vi "Fix BD Size.vi"(8 "error in (no error)":errorcluster, 11 "vi ref":refnum<vi>) -> (0 "error out":errorcluster, 3 "vi ref (dup)":refnum<vi>)   [LabVIEW 2021]
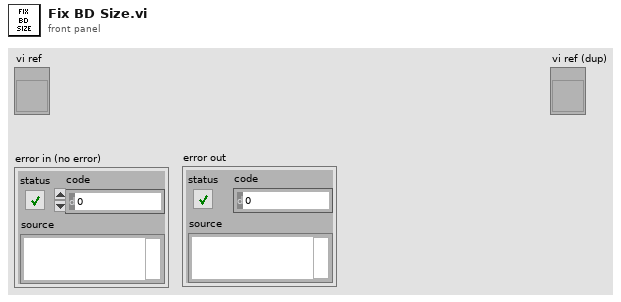
[diagram p1: front panel]
types:
  T1 = cluster{"min x":i32, "min y":i32, "max x":i32, "max y":i32}
  T2 = typedef "LVRectTypeDef.ctl" = cluster{"Left":i16, "Top":i16, "Right":i16, "Bottom":i16}
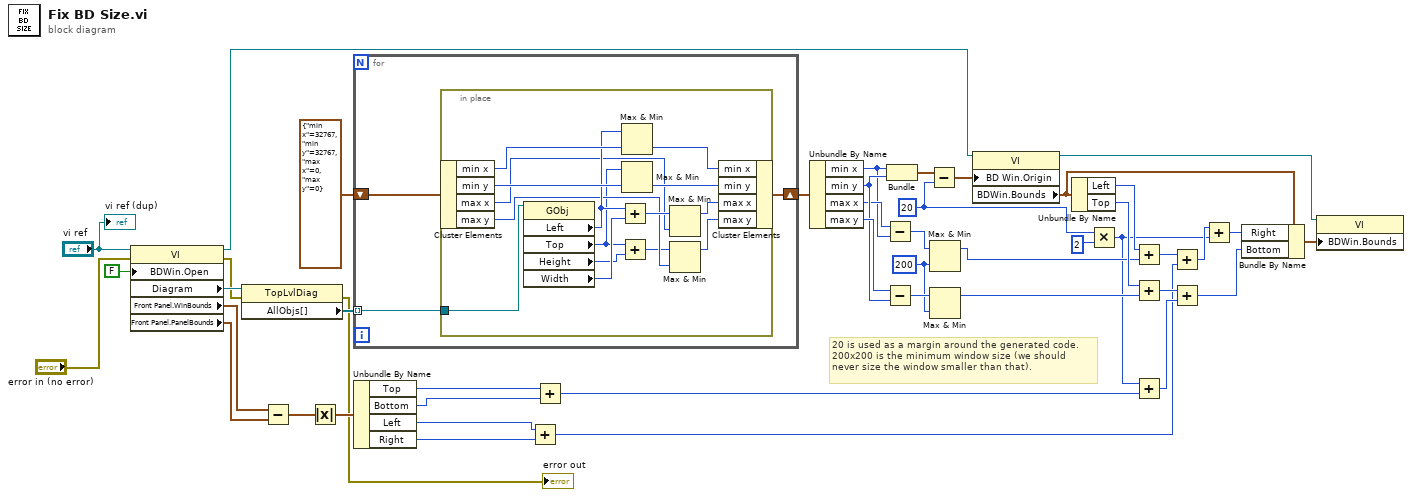
[diagram p0: block diagram]
diagram:
  w11 = 20 ("y")
  w24 = 200 ("y")
  # "20 is used as a margin around the generated code.\n200x200 is the minimum window size (we should\nnever size the window smaller than that)."
  n1 = property class="VI"(reference="vi ref", error in="error in (no error)", "BDWin.Open"=FALSE ("Block Diagram Window:Open")) -> (reference out=w40:refnum<vi>, error out=w2:errorcluster, "Diagram"=w43:refnum<vi>, "Front Panel.WinBounds"=w20:T2, "Front Panel.PanelBounds"=w19:T2)
  n2 = property class="TopLvlDiag"(reference=w43, error in=w2) -> (error out=→"error out":errorcluster, "AllObjs[]"=w42:refnum<vi>[])  [unwired: 1 out]
  n3 = Subtract(x=w20, y=w19) -> (x-y=w9:T2)
  n4 = Absolute Value(x=w9) -> (abs(x)=w8:T2)
  n5 = for {
    tunnel: w42 -> [w47] mode=indexing
    shift-right: [w46] -> w39
    shift-left: T1 {"min x"=32767, "min y"=32767, "max x"=0, "max y"=0} -> [w48]
    n6 = in-place {
      in-place-border: w47 -> [w63]
      n7 = in-place-cluster #1(w48) -> ("min x"=w62:i32, "min y"=w60:i32, "max x"=w55:i32, "max y"=w53:i32)
      n8 = property class="GObj"(reference=w63) -> ("Left"=w58:i32, "Top"=w52:i32, "Height"=w51:u32, "Width"=w57:u32)  [unwired: 1 in, 2 out]
      n9 = Add(x=w58, y=w57) -> (x+y=w56:u32)
      n10 = Add(x=w52, y=w51) -> (x+y=w50:u32)
      n11 = Max & Min(x=w58, y=w62) -> (min(x,y)=w61:i32)  [unwired: 1 out]
      n12 = Max & Min(x=w52, y=w60) -> (min(x,y)=w59:i32)  [unwired: 1 out]
      n13 = Max & Min(x=w56, y=w55) -> (max(x,y)=w54:u32)  [unwired: 1 out]
      n14 = Max & Min(x=w50, y=w53) -> (max(x,y)=w49:u32)  [unwired: 1 out]
      n15 = in-place-cluster #1("min x"=w61, "min y"=w59, "max x"=w54, "max y"=w49) -> (w46:T1)
    }
  }
  n16 = Unbundle By Name(w8) -> ("Top"=w7:i16, "Bottom"=w6:i16, "Left"=w5:i16, "Right"=w4:i16)
  n17 = Add(x=w5, y=w4) -> (x+y=w15:i16)
  n18 = Add(x=w7, y=w6) -> (x+y=w17:i16)
  n19 = Unbundle By Name(w39) -> ("min x"=w35:i32, "min y"=w37:i32, "max x"=w36:i32, "max y"=w38:i32)
  n20 = Subtract(x=w36, y=w35) -> (x-y=w27:i32)
  n21 = Subtract(x=w38, y=w37) -> (x-y=w25:i32)
  n22 = Bundle("min x"=w35, "min y"=w37) -> (w22:cluster{"min x":i32, "min y":i32})  [unwired: 1 in]
  n23 = Subtract(x=w22, y=w11) -> (x-y=w21:cluster{"min x":i32, "min y":i32})
  n24 = Max & Min(x=w27, y=w24) -> (max(x,y)=w26:i32)  [unwired: 1 out]
  n25 = Max & Min(x=w25, y=w24) -> (max(x,y)=w23:i32)  [unwired: 1 out]
  n26 = property class="VI"(reference=w40, "BD Win.Origin"=w21) -> (reference out=w31:refnum<vi>, "BDWin.Bounds"=w32:T2)  [unwired: 1 in, 1 out]
  n27 = Unbundle By Name(w32) -> ("Left"=w34:i16, "Top"=w33:i16)
  n28 = Multiply(x=w11, y=2) -> (x*y=w10:i32)
  n29 = Add(x=w34, y=w26) -> (x+y=w16:i32)
  n30 = Add(x=w33, y=w23) -> (x+y=w29:i32)
  n31 = Add(x=w10, y=w17) -> (x+y=w18:i32)
  n32 = Add(x=w16, y=w15) -> (x+y=w14:i32)
  n33 = Add(x=w29, y=w18) -> (x+y=w28:i32)
  n34 = Add(x=w14, y=w10) -> (x+y=w13:i32)
  n35 = Bundle By Name(cluster=w32, "Right"=w13, "Bottom"=w28) -> (w30:T2)
  n36 = property class="VI"(reference=w31, "BDWin.Bounds"=w30) -> ()  [unwired: 1 in, 2 out]
  "vi ref (dup)" <- "vi ref"
